vi "836_MultiCameraSend Images To PC Loop.vi"(8 "error in (no error)":errorcluster, 10 "port":u16=1180, 11 "CameraDevRef":T1) -> ()   [LabVIEW 2015]
doc: "This VI is used to send images to the dashboard using the second enet port on the 8 slot controller. This is provided for compatibility, but is higher overhead than using the Camera MJPG approach.\n\nThis software is licensed. Open the labview\\readme\\WPI Robotics Library Open Source License.txt file for more information."
uses:
  <vilib>/Rock Robotics/WPI/Camera/WPI_CameraDevRef.ctl
  <vilib>/Rock Robotics/SystemInterfaces/NetworkCommunication/NetComm_UsageReport_ResourceType.ctl
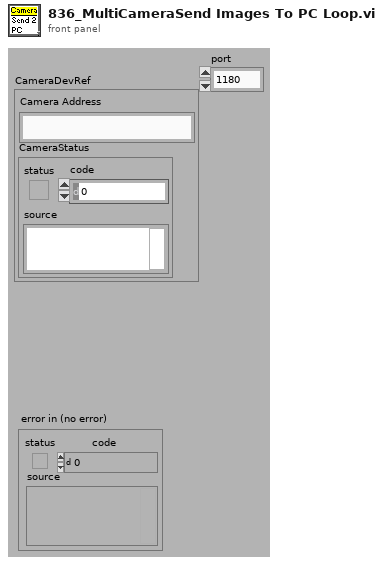
[diagram p1: front panel]
types:
  T1 = typedef "WPI_CameraDevRef.ctl" = cluster{"Camera Address":string, "CameraStatus":errorcluster}
  T2 = cluster{"fps":i32, "compression":i32, "compression 2":i32}
  T3 = typedef "NetComm_UsageReport_ResourceType.ctl" = enum8{"Controller", "Module", "Language", "CANPlugin", "Accelerometer", "ADXL345", "AnalogChannel", "AnalogTrigger", "AnalogTriggerOutput", "CANJaguar", "Compressor", "Counter", "Dashboard", "DigitalInput", "DigitalOutput", "DriverStationCIO", "DriverStationEIO", "DriverStationLCD", "Encoder", "GearTooth", "Gyro", "I2C", "Framework", "Jaguar", "Joystick", "Kinect", "KinectStick", "PIDController", "Preferences", "PWM", "Relay", "RobotDrive", "SerialPort", "Servo", "Solenoid", "SPI", "Task", "Ultrasonic", "Victor", "Button", "Command", "AxisCamera", "PCVideoServer", "SmartDashboard", "Talon", "HiTechnicColorSensor", "HiTechnicAccel", "HiTechnicCompass", "SRF08", "AnalogOutput", "Victor SP", "Talon SRX", "CAN Talon SRX", "ADXL362 Accel", "ADXRS450 Gyro", "Rev SPARK", "Mindsensors SD540", "Digital Filter"}
  T4 = enum16{"Update Mode", "Get Image", "Get Image Data"}
  T5 = typedef "Image Type" = u32
  T6 = typedef "IMAQ Image.ctl" = refnum<image>
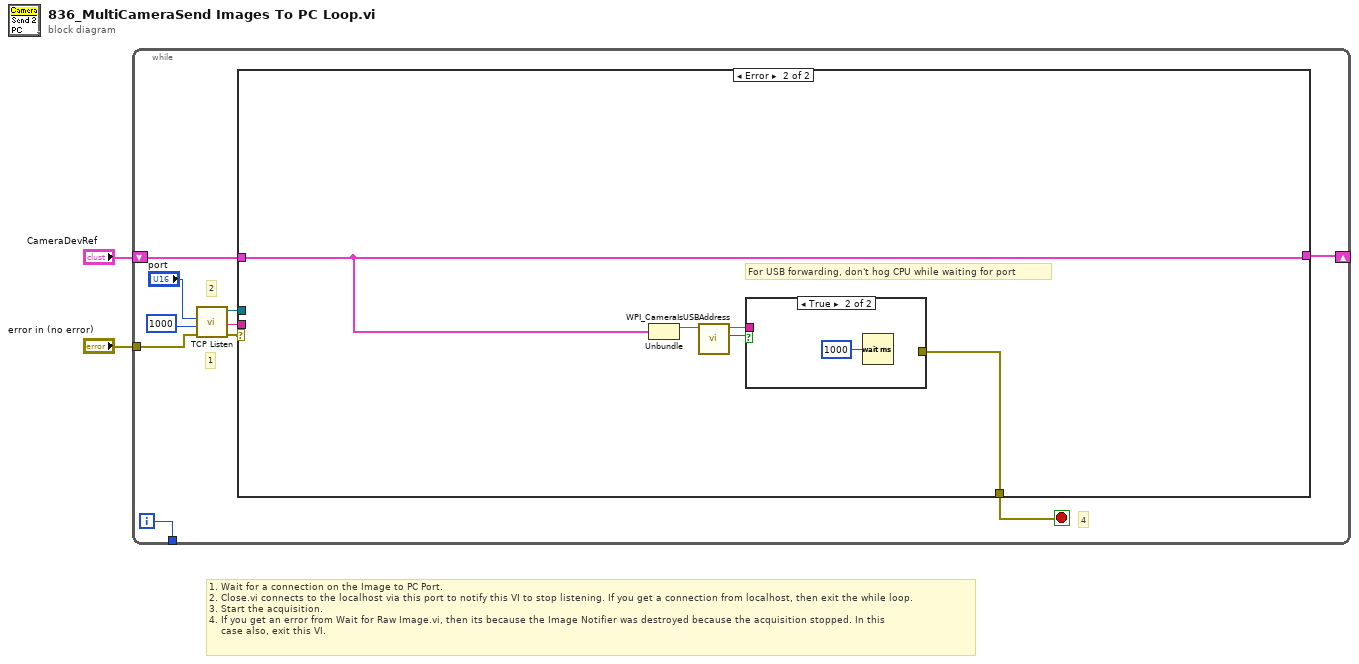
[diagram p0: block diagram]
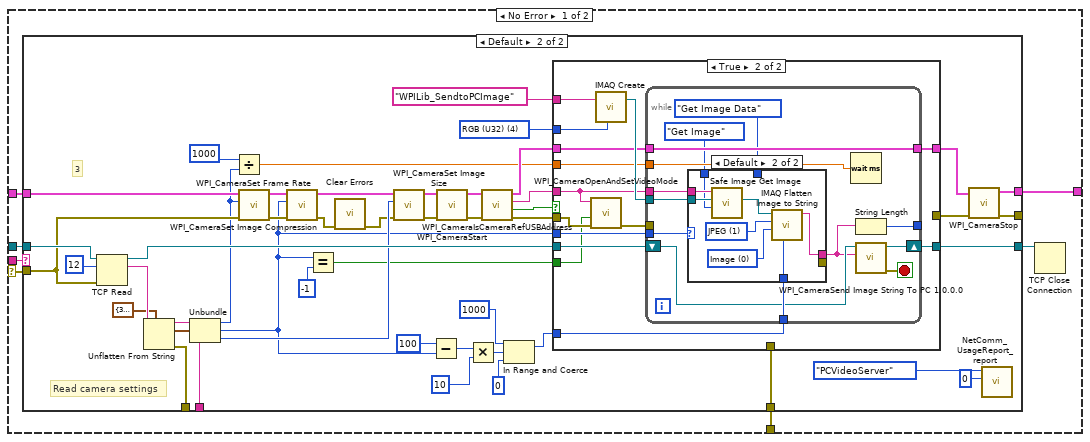
[diagram p2: hidden frame]
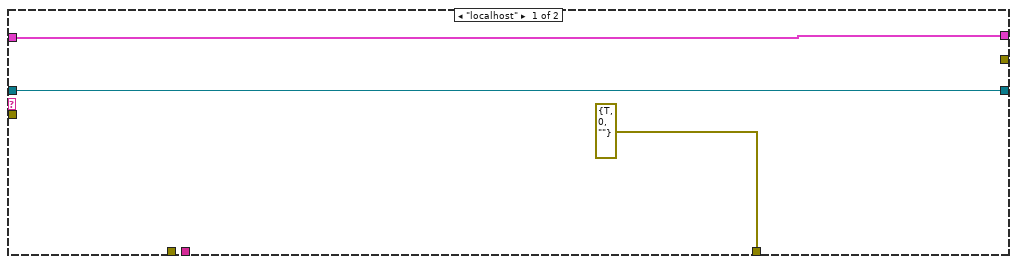
[diagram p3: hidden frame]
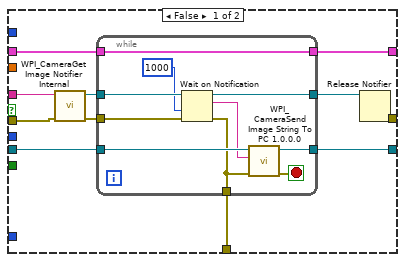
[diagram p4: hidden frame]
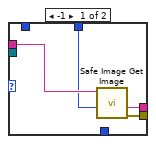
[diagram p5: hidden frame]
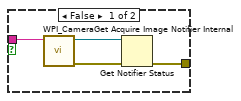
[diagram p6: hidden frame]
diagram:
  # "1. Wait for a connection on the Image to PC Port.\n2. Close.vi connects to the localhost via this port to notify this VI to stop listening. If you get a connection from localhost, then exit the while loop.\n3. Start the acquisition.\n4. If you get an error from Wait for Raw Image.vi, then its because the Image Notifier was destroyed because the acquisition stopped. In this\n    case also, exit this VI."
  n1 = while {
    tunnel: "error in (no error)" -> [w9]
    shift-right: [w12] -> _
    shift-left: "CameraDevRef" -> [w10]
    tunnel: [w3] -> _
    i -> [w3]
    stop <- w7 stop-if-true
    # "4"
    # "1"
    # "2"
    n2 = call <vilib>:"TCP Listen.vi"("error in (no error)"=w9, "timeout ms (wait forever: -1)"=u16 1000 ("port"), "port"="port") -> ("error out"=w5:errorcluster, "remote address"=w11:string, "connection ID"=w8:refnum<k5>)  [unwired: 1 in, 5 out]
    n3 = case shown="Error" w5 {
      selector: w5 -> [w13 _]
      tunnel: [w19 w133] -> w12
      tunnel: w11 -> [w18 _]
      tunnel: w10 -> [w17 w133]
      tunnel: w8 -> [w16 _]
      tunnel: [w15 w134] -> w7
      frame No Error {
        n4 = case shown="Default" w18 {
          tunnel: [w22 w67] -> w19
          tunnel: w17 -> [w22 w49]
          tunnel: w13 -> [_ w45]
          tunnel: w16 -> [w20 w53]
          tunnel: [errorcluster {"status"=TRUE, "code"=0, "source"=""} ("error out 2") w69] -> w15
          tunnel: [w20 w68] -> w14
          tunnel: [_ w66] -> _
          tunnel: [_ w24] -> _
          tunnel: [_ w23] -> _
          frame "localhost" {
          }
          frame Default {
            w60 = T5 4 items=["Grayscale (U8)", "Grayscale (I16)", "Grayscale (SGL)", "Complex (CSG)", "RGB (U32)", "HSL (U32)", "RGB (U64)", "Grayscale (U16)"] ("Image Type")
            # "Read camera settings"
            # "3"
            n5 = TCP Read(connection ID=w53, bytes to read=12, error in (no error)=w45) -> (connection ID out=w52:refnum<k5>, data out=w50:string)  [unwired: 2 in, 1 out]
            n6 = Unflatten From String(type=T2 {"fps"=30, "compression"=32, "compression 2"=32} ("Camera Settings"), binary string=w50) -> (rest of the binary string=w23:string, value=w42:T2, error out=w24:errorcluster)  [unwired: 3 in]
            n7 = Unbundle(w42) -> ("fps"=w39:i32, "compression"=w28:i32, "compression 2"=w41:i32)
            n8 = Divide(x=u16 1000 ("port"), y=w39) -> (x/y=w38:dbl)
            n9 = call <vilib>:"WPI_CameraSet Frame Rate.vi"("error in (no error)"=w45, "Frame Rate (fps)"=w39, "CameraDevRef"=w49) -> ("error out"=w44:errorcluster, "CameraDevRef Out"=w48:T1)  [unwired: 7 in]
            n10 = call <vilib>:"WPI_CameraSet Image Compression.vi"("error in (no error)"=w44, "Compression"=w28, "CameraDevRef"=w48) -> ("error out"=w26:errorcluster, "CameraDevRef Out"=w47:T1)  [unwired: 7 in]
            n11 = Equal?(x=w28, y=-1) -> (x = y?=w27:bool)
            n12 = call <vilib>:"Clear Errors.vi"("error in (no error)"=w26) -> ("error out"=w25:errorcluster)  [unwired: 5 in, 1 out]
            n13 = call <vilib>:"WPI_CameraSet Image Size.vi"("error in (no error)"=w25, "Image Size"=w41, "CameraDevRef"=w47) -> ("error out"=w43:errorcluster, "CameraDevRef Out"=w46:T1)  [unwired: 7 in]
            n14 = Subtract(x=100, y=w28) -> (x-y=w33:i32)
            n15 = call <vilib>:"WPI_CameraStart.vi"("error in (no error)"=w43, "CameraDevRef"=w46) -> ("error out"=w57:errorcluster, "CameraDevRef"=w55:T1)  [unwired: 8 out]
            n16 = Multiply(x=w33, y=10) -> (x*y=w35:i32)
            n17 = call <vilib>:"WPI_CameraIsCameraRefUSBAddress.vi"("error in (no error)"=w57, "CameraDevRef"=w55) -> ("error out"=w56:errorcluster, "USB?"=w58:bool, "Camera Address Out"=w59:string, "CameraDevRef out"=w54:T1)  [unwired: 6 in]
            n18 = In Range and Coerce(upper limit=1000, x=w35, lower limit=0) -> (coerced(x)=w31:i32)  [unwired: 1 out]
            n19 = case shown="True" w58 {
              tunnel: w52 -> [w80 w104]
              tunnel: [w79 _] -> w69
              tunnel: [w78 w103] -> w68
              tunnel: w56 -> [w77 w94]
              tunnel: w59 -> [w75 w93]
              tunnel: [w74 w98] -> w65
              tunnel: w54 -> [w73 w99]
              tunnel: [w71 _] -> w64
              tunnel: "WPILib_SendtoPCImage" -> [_ w101]
              tunnel: w60 -> [_ w100]
              tunnel: w31 -> [_ w97]
              tunnel: w38 -> [_ w96]
              tunnel: w28 -> [_ w95]
              tunnel: w27 -> [_ w91]
              frame False {
                n20 = call <vilib>:"WPI_CameraGet Image Notifier Internal.vi"("error in (no error)"=w77, "Camera Address"=w75) -> ("error out"=w76:errorcluster, "Image Notifier"=w72:refnum<notifier>)  [unwired: 8 out]
                n21 = while {
                  tunnel: w76 -> [w86]
                  tunnel: w80 -> [w90]
                  tunnel: [w83] -> w79
                  tunnel: [w88] -> w78
                  tunnel: [w87] -> w74
                  tunnel: w73 -> [w87]
                  tunnel: w72 -> [w85]
                  tunnel: [w81] -> w70
                  stop <- w89 stop-if-true
                  n22 = Wait on Notification(notifier=w85, timeout in ms (-1)=1000 ("Timeout in ms (-1)"), error in (no error)=w86) -> (notifier out=w81:refnum<notifier>, notification=w84:string, error out=w83:errorcluster)  [unwired: 2 out]
                  n23 = call <vilib>:"WPI_CameraSend Image String To PC 1.0.0.0.vi"("error in (no error)"=w83, "String"=w84, "TCP Connection ID"=w90) -> ("error out"=w89:errorcluster, "TCP Connection ID out"=w88:refnum<k5>)  [unwired: 7 out]
                }
                n24 = Release Notifier(notifier=w70) -> (error out=w71:errorcluster)  [unwired: 1 in, 3 out]
              }
              frame True {
                n25 = call <vilib>:"WPI_CameraOpenAndSetVideoMode.vi"("error in (no error)"=w94, "USB JPEG"=w91, "Camera Address Out"=w93) -> ("error out"=w92:errorcluster)  [unwired: 8 in]
                n26 = call "IMAQ Create"("Image Name"=w101, "Image Type"=w100) -> ("New Image"=w102:T6)  [unwired: 3 in, 1 out]
                n27 = while {
                  tunnel: w93 -> [w116]
                  shift-right: [w117] -> w103
                  shift-left: w104 -> [w110]
                  tunnel: w102 -> [w115]
                  tunnel: [w113] -> w98
                  tunnel: w99 -> [w113]
                  tunnel: w97 -> [w112]
                  tunnel: w96 -> [w111]
                  tunnel: [w108] -> _
                  tunnel: w95 -> [w107]
                  tunnel: w92 -> [_]
                  stop <- w114 stop-if-true
                  n28 = case shown="Default" w107 {
                    tunnel: [w120 w129] -> w109
                    tunnel: w116 -> [w121 w125]
                    tunnel: w115 -> [_ w124]
                    tunnel: w112 -> [_ w126]
                    tunnel: [w119 _] -> _
                    tunnel: T4."Get Image Data" ("Operation") -> [w118 _]
                    tunnel: T4."Get Image" ("Operation") -> [_ w122]
                    frame -1 {
                      n29 = call <vilib>:"Safe Image Get Image.vi"("Operation"=w118, "Session In"=w121) -> ("error out"=w119:errorcluster, "Image Data String"=w120:string)  [unwired: 6 in, 2 out]
                    }
                    frame Default {
                      w127 = 0 items=["Image", "Image and Vision Info", "Reference to Image"] ("Type of Flatten (Image and Vision Info)")
                      w128 = 1 items=["None", "JPEG", "PACKED BINARY"] ("Compression (None)")
                      n30 = call <vilib>:"Safe Image Get Image.vi"("Operation"=w122, "Image In"=w124, "Session In"=w125) -> ("Image Out"=w123:T6)  [unwired: 5 in, 3 out]
                      n31 = call "IMAQ Flatten Image to String"("Quality (750)"=w126, "Type of Flatten (Image and Vision Info)"=w127, "Compression (None)"=w128, "Image"=w123) -> ("Data String"=w129:string)  [unwired: 6 in, 1 out]
                    }
                  }
                  n32 = Wait (ms)(milliseconds to wait=w111) -> ()  [unwired: 1 out]
                  n33 = String Length(string=w109) -> (length=w108:i32)
                  n34 = call <vilib>:"WPI_CameraSend Image String To PC 1.0.0.0.vi"("String"=w109, "TCP Connection ID"=w110) -> ("error out"=w114:errorcluster, "TCP Connection ID out"=w117:refnum<k5>)  [unwired: 1 in, 7 out]
                }
              }
            }
            n35 = call <vilib>:"WPI_CameraStop.vi"("error in (no error)"=w64, "CameraDevRef"=w65) -> ("error out"=w66:errorcluster, "CameraDevRef"=w67:T1)  [unwired: 8 out]
            n36 = call <vilib>:"NetComm_UsageReport_report.vi"("Instance Number"=u8 0, "Resource Type"=NetComm_UsageReport_ResourceType."PCVideoServer") -> ()  [unwired: 10 in]
          }
        }
        n37 = TCP Close Connection(connection ID=w14) -> ()  [unwired: 1 in, 3 out]
      }
      frame Error {
        # "For USB forwarding, don't hog CPU while waiting for port"
        n38 = Unbundle(w133) -> ("Camera Address"=w132:string)  [unwired: 1 out]
        n39 = call <vilib>:"WPI_CameraIsUSBAddress.vi"("Camera Address In"=w132) -> ("USB?"=w130:bool, "Camera Address Out"=w131:string)  [unwired: 8 in, 1 out]
        n40 = case shown="True" w130 {
          tunnel: [w138 _] -> w134
          tunnel: w131 -> [w135 _]
          frame False {
            n41 = call <vilib>:"WPI_CameraGet Acquire Image Notifier Internal.vi"("Camera Address"=w135) -> ("error out"=w136:errorcluster, "Acquire Image Notifier"=w137:refnum<notifier>)  [unwired: 1 in, 8 out]
            n42 = Get Notifier Status(notifier=w137, error in (no error)=w136) -> (error out=w138:errorcluster)  [unwired: 4 out]
          }
          frame True {
            n43 = Wait (ms)(milliseconds to wait=u32 1000) -> ()  [unwired: 1 out]
          }
        }
      }
    }
  }
